vi "Add Test Result.vi"(8 "error in (no error)":errorcluster, 10 "Test Result":refnum<class "Test Result.lvclass">, 11 "ResultTree in":refnum<class "Result Tree.lvclass">) -> (0 "error out":errorcluster, 3 "ResultTree out":refnum<class "Result Tree.lvclass">)   [LabVIEW 2017, in "Result Tree.lvclass"]
doc: "Adds the specified test results to the tree."
uses:
  Result Tree.lvclass
  Test Result/Test Result.lvclass
  Test Result/Test Result.lvclass/Test Result.ctl
  Test Case/Test Case.lvclass/Test Case.ctl
  Test Result/Get Test Case.vi
  Test Result/Get Failure Message.vi
  Test Result/Get Outcome.vi
  Test Result/Get Start Time.vi
  Test Result/Get End Time.vi
  Test Case/Get Qualified Name.vi
  Test Case/Test Case.lvclass
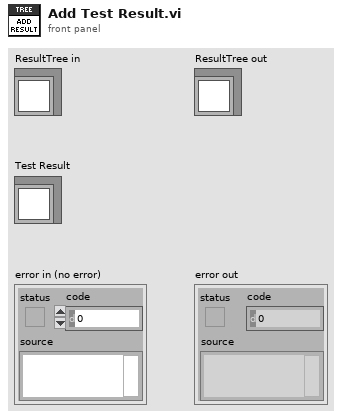
[diagram p1: front panel]
types:
  T1 = typedef "Test Outcome.ctl" = enum16{"None", "Passed", "Failed"}
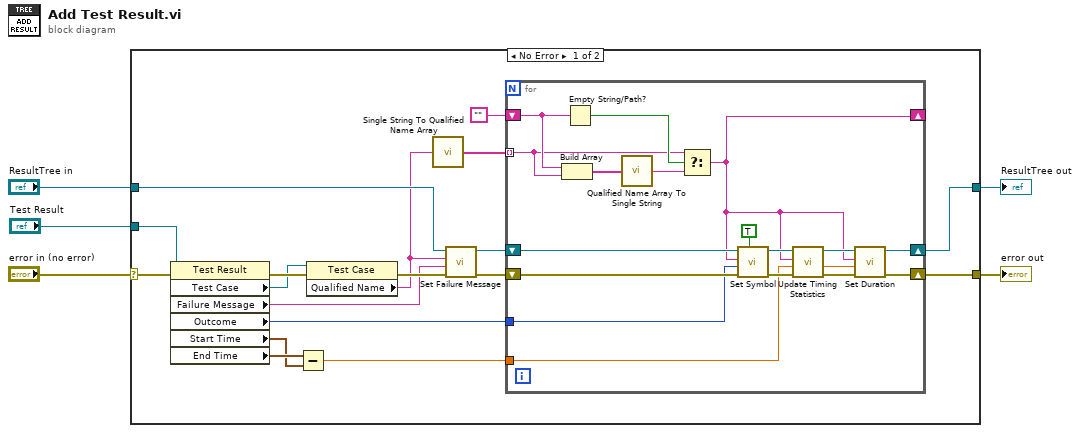
[diagram p0: block diagram]
diagram:
  n1 = case shown="No Error" "error in (no error)" {
    selector: "error in (no error)" -> [w22 w43]
    tunnel: [w23 w43] -> w4
    tunnel: [w19 w42] -> w2
    tunnel: "ResultTree in" -> [w20 w42]
    tunnel: "Test Result" -> [w21 _]
    frame No Error {
      n2 = property class="Test Result"(reference=w21, error in=w22) -> (error out=w18:errorcluster, "Test Case"=w17:refnum<class "Test Case.lvclass">, "Failure Message"=w6:string, "Outcome"=w16:T1, "Start Time"=w12:timestamp, "End Time"=w13:timestamp)  [unwired: 1 out]
      n3 = Subtract(x=w13, y=w12) -> (x-y=w11:dbl)
      n4 = property class="Test Case"(reference=w17, error in=w18) -> (error out=w10:errorcluster, "Qualified Name"=w7:string)  [unwired: 1 out]
      n5 = call <vilib>:"Single String To Qualified Name Array.vi"("Fully Qualified String"=w7) -> ("Fully Qualified Array"=w15:string[])
      n6 = call "Set Failure Message.vi"("error in (no error)"=w10, "Error Message"=w6, "Tag Name"=w7, "ResultTree in"=w20) -> ("error out"=w9:errorcluster, "ResultTree out"=w8:refnum<class "Result Tree.lvclass">)  [unwired: 6 in]
      n7 = for {
        tunnel: w16 -> [w39]
        shift-right: [w33] -> w23
        shift-left: w9 -> [w41]
        tunnel: w15 -> [w36] mode=indexing
        shift-right: [w25] -> _
        shift-left: "" -> [w37]
        shift-right: [w32] -> w19
        shift-left: w8 -> [w40]
        tunnel: w11 -> [w24]
        n8 = Build Array(w37, w36) -> (w35:string[])
        n9 = Empty String/Path?(string/path=w37) -> (empty?=w38:bool)
        n10 = call <vilib>:"Qualified Name Array To Single String.vi"("Fully Qualified Array"=w35) -> ("Fully Qualified String"=w34:string)
        n11 = Select(t=w36, s=w38, f=w34) -> (s? t:f=w25:string)
        n12 = call "Set Symbol.vi"("Skip If Worse (F)"=TRUE, "error in (no error)"=w41, "Test Outcome"=w39, "Tag Name"=w25, "ResultTree in"=w40) -> ("error out"=w28:errorcluster, "ResultTree out"=w30:refnum<class "Result Tree.lvclass">)  [unwired: 5 in]
        n13 = call "Update Timing Statistics.vi"("error in (no error)"=w28, "Time to Add"=w24, "Qualified Name"=w25, "ResultTree in"=w30) -> ("error out"=w27:errorcluster, "Total Time"=w26:dbl, "ResultTree out"=w29:refnum<class "Result Tree.lvclass">)  [unwired: 5 in]
        n14 = call "Set Duration.vi"("error in (no error)"=w27, "Duration [s]"=w26, "Tag Name"=w25, "ResultTree in"=w29) -> ("error out"=w33:errorcluster, "ResultTree out"=w32:refnum<class "Result Tree.lvclass">)  [unwired: 6 in]
      }
    }
    frame Error {
    }
  }
  "error out" <- w4
  "ResultTree out" <- w2
